vi "Test Append Row Values on Closed File.vi"(11 "Test Case In":refnum<class "Test Open Xml.lvclass">) -> (0 "error out":errorcluster, 3 "Test Case Out":refnum<class "Test Open Xml.lvclass">)   [LabVIEW 2020, in "Test Open Xml.lvclass"]
uses:
  Test Open Xml.lvclass
  <vilib>/Astemes/LUnit/Test Case.lvclass/Test Case.ctl
  <vilib>/Comparison/Equal/Equal Functor/Equal Functor.lvclass
  Test Open Xml.lvclass/Test Open Xml.ctl
  Source/Open Xml.lvlib
  <vilib>/Astemes/LUnit/Test Case.lvclass
  C:/Program Files/National Instruments/LabVIEW 2025/vi.lib/Astemes/LUnit/Test Case.lvclass
  C:/Program Files/National Instruments/LabVIEW 2025/vi.lib/Astemes/LUnit/LUnit Runnable.lvclass
  D:/git/Open-Xml-LabVIEW/Test Open Xml/Test Open Xml.lvclass
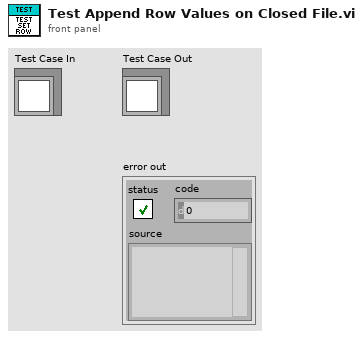
[diagram p1: front panel]
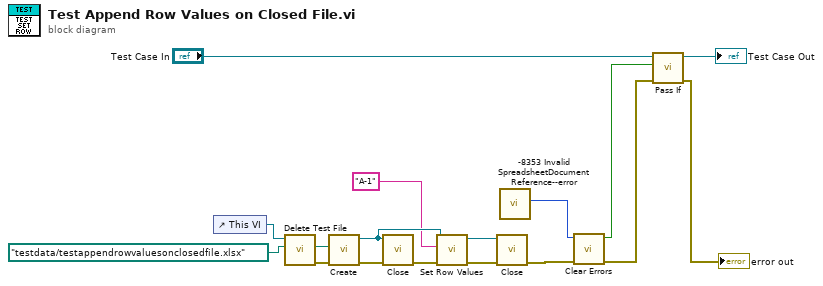
[diagram p0: block diagram]
diagram:
  n1 = control-ref of="This VI"() -> (w11:refnum<vi>)
  n2 = call "Delete Test File.vi"("name or relative path"=path "testdata/testappendrowvaluesonclosedfile.xlsx", "VI in"=w11) -> ("error out"=w12:errorcluster, "deleted path"=w9:path)  [unwired: 8 in]
  n3 = call "Create.vi"("error in"=w12, "Path"=w9) -> ("error out"=w13:errorcluster, "SpreadsheetDoc"=w14:refnum<k24>)  [unwired: 8 in]
  n4 = call "Close.vi"("error in"=w13, "SpreadsheetDoc"=w14) -> ("error out"=w5:errorcluster)  [unwired: 9 in]
  n5 = call "Set Row Values.vi"("error in"=w5, "Cell Address"="A-1", "SpreadsheetDoc"=w14) -> ("error out"=w8:errorcluster, "SpreadsheetDoc out"=w7:refnum<k24>)  [unwired: 7 in]
  n6 = call "Close.vi"("error in"=w8, "SpreadsheetDoc"=w7) -> ("error out"=w4:errorcluster)  [unwired: 9 in]
  n7 = call "-8353 Invalid SpreadsheetDocument Reference--error.vi"() -> ("Error Code"=w2:i32)  [unwired: 10 in, 1 out]
  n8 = call <vilib>:"Clear Errors.vi"("error in (no error)"=w4, "specific error code to clear (0: all)"=w2) -> ("error out"=w3:errorcluster, "specific error cleared?"=w1:bool)  [unwired: 4 in]
  n9 = call <vilib>:"Pass If.vi"("error in (no error)"=w3, "Pass?"=w1, "LUnit Test Case In"="Test Case In") -> ("error out"=→"error out":errorcluster, "LUnit Test Case Out"=→"Test Case Out":refnum<class "Test Open Xml.lvclass">)  [unwired: 7 in]
